vi "StopSignal-StopAllInOrder.vi"(7 "reverse?":bool=TRUE, 8 "error in (no error)":errorcluster, 9 "timeout(ms)":i32=5000, 10 "reason(\"\")":string, 11 "StopSignal":T1) -> (0 "error out":errorcluster, 3 "StopSignal(dup)":T1)   [LabVIEW 2017, in "StopSignal.lvlib"]
uses:
  StopSignal.lvlib
  Typedef/StopSignal.ctl
  Typedef/Action.ctl
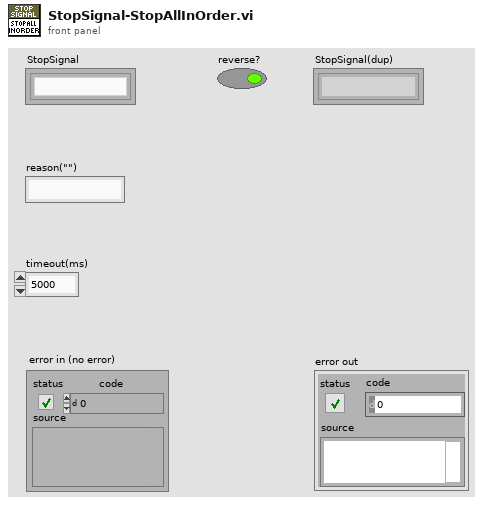
[diagram p1: front panel]
types:
  T1 = typedef "StopSignal.lvlib/StopSignal.ctl" = refnum<k1>
  T2 = typedef "StopSignal.lvlib/Action.ctl" = enum16{"Counter-Increment", "Counter-Decrement", "Counter-Name", "Get-All-Signals-Inorder", "Get-Stop-Signal-Lib"}
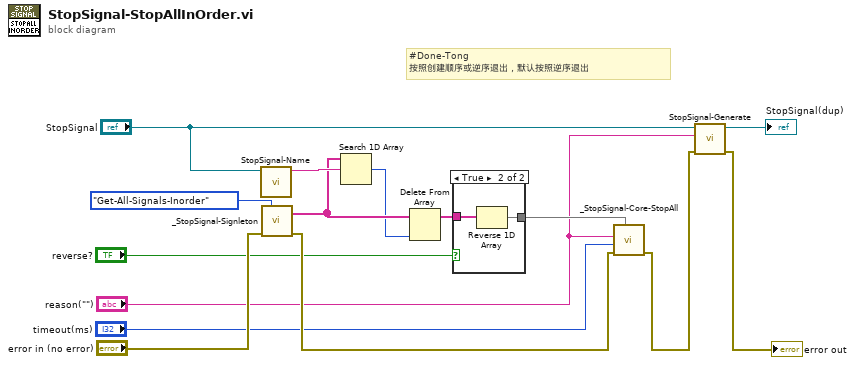
[diagram p0: block diagram]
diagram:
  # "#Done-Tong\n按照创建顺序或逆序退出，默认按照逆序退出"
  n1 = call "StopSignal-Name.vi"("StopSignal"="StopSignal") -> ("name"=w8:string)  [unwired: 9 in, 1 out]
  n2 = call "_StopSignal-Signleton.vi"("Action"=Action."Get-All-Signals-Inorder", "error in"="error in (no error)") -> ("AllSignalsInorder"=w7:string[], "error out"=w14:errorcluster)  [unwired: 8 in, 4 out]
  n3 = Search 1D Array(1D array=w7, element=w8) -> (index of element=w6:i32)  [unwired: 1 in]
  n4 = Delete From Array(array=w7, index=w6) -> (array with subset deleted=w5:string[])  [unwired: 1 in, 1 out]
  n5 = case shown="True" "reverse?" {
    tunnel: w5 -> [w16 w18]
    tunnel: [w16 w17] -> w3
    frame False {
    }
    frame True {
      n6 = Reverse 1D Array(array=w18) -> (reversed array=w17:string[])
    }
  }
  n7 = call "_StopSignal-Core-StopAll.vi"("name(\"\")"=w3, "error in (no error)"=w14, "timeout(ms)"="timeout(ms)", "reason(\"\")"="reason(\"\")") -> ("error out"=w12:errorcluster)  [unwired: 7 in]
  n8 = call "StopSignal-Generate.vi"("error in (no error)"=w12, "reason(\"\")"="reason(\"\")", "StopSignal"="StopSignal") -> ("error out"=→"error out":errorcluster, "StopSignal(dup)"=→"StopSignal(dup)":T1)  [unwired: 7 in]
